vi "exponential.vi"(8 "n":dbl, 10 "x":dbl) -> (2 "exp(x)":dbl)   [LabVIEW 2019]
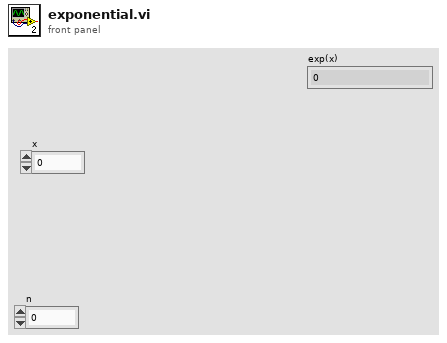
[diagram p1: front panel]
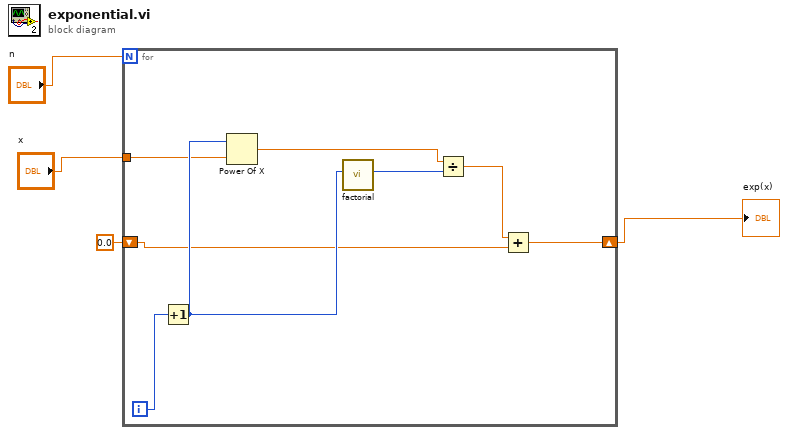
[diagram p0: block diagram]
diagram:
  n1 = for {
    N: "n" -> [_]
    tunnel: "x" -> [w7]
    shift-right: [w6] -> w1
    shift-left: 0.0 -> [w5]
    i -> [w11]
    n2 = Increment(x=w11) -> (x+1=w8:i32)
    n3 = Power Of X(1:w7, 2:w8) -> (0:w10:dbl)
    n4 = call "factorial.vi"("n"=w8) -> ("n!"=w12:u64)  [unwired: 10 in]
    n5 = Divide(x=w10, y=w12) -> (x/y=w9:dbl)
    n6 = Add(x=w9, y=w5) -> (x+y=w6:dbl)
  }
  "exp(x)" <- w1
